vi "F510-X.vi"(8 "error in (no error)":errorcluster, 10 "Deadzone Scale Cluster":cluster{"Scale":dbl, "Deadzone":dbl}={"Scale"=1.0, "Deadzone"=0.1}, 11 "refnum name":string) -> (0 "error out":errorcluster, 1 "Right Stick":cluster{"X":dbl, "Y":dbl}, 2 "Left Stick":cluster{"X":dbl, "Y":dbl}, 3 "JoystickDevRef":T2, 4 "Buttons":T1, 5 "Triggers":cluster{"Left":dbl, "Right":dbl}, 6 "D-Pad Buttons":T4)   [LabVIEW 2016]
uses:
  <vilib>/Rock Robotics/WPI/Joystick/WPI_JoystickDevRef.ctl
  <vilib>/Rock Robotics/WPI/Joystick/WPI_JoystickDeviceEnum.ctl
  <vilib>/Rock Robotics/WPI/Utilities/WPI_GetSetVariantRefNum.vi
panel:
  in  "Smooth Control (T)":bool=TRUE
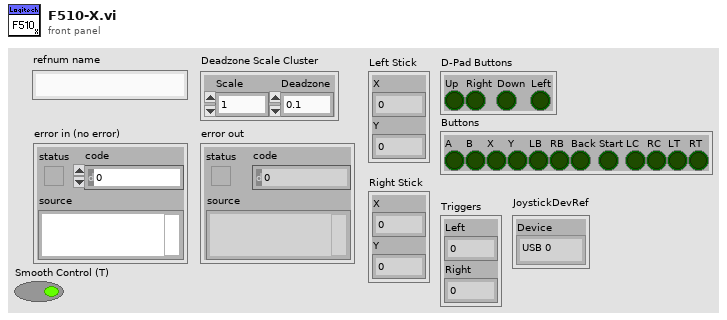
[diagram p1: front panel]
types:
  T1 = cluster{"A":bool, "B":bool, "X":bool, "Y":bool, "LB":bool, "RB":bool, "Back":bool, "Start":bool, "LC":bool, "RC":bool, "LT":bool, "RT":bool}
  T2 = typedef "WPI_JoystickDevRef.ctl" = cluster{"Device":T3}
  T3 = typedef "WPI_JoystickDeviceEnum.ctl" = enum16{"USB 0", "USB 1", "USB 2", "USB 3", "USB 4", "USB 5"}
  T4 = cluster{"Up":bool, "Right":bool, "Down":bool, "Left":bool}
  T5 = cluster{"[0]":dbl, "[1]":dbl, "[2]":dbl, "[3]":dbl, "[4]":dbl, "[5]":dbl}
  T6 = cluster{"Buttons[0]":bool, "Buttons[1]":bool, "Buttons[2]":bool, "Buttons[3]":bool, "Buttons[4]":bool, "Buttons[5]":bool, "Buttons[6]":bool, "Buttons[7]":bool, "Buttons[8]":bool, "Buttons[9]":bool}
  T7 = cluster{"Up":bool, "Down":bool, "Left":bool, "Right":bool}[]
  T8 = cluster{"Up":bool, "Down":bool, "Left":bool, "Right":bool}
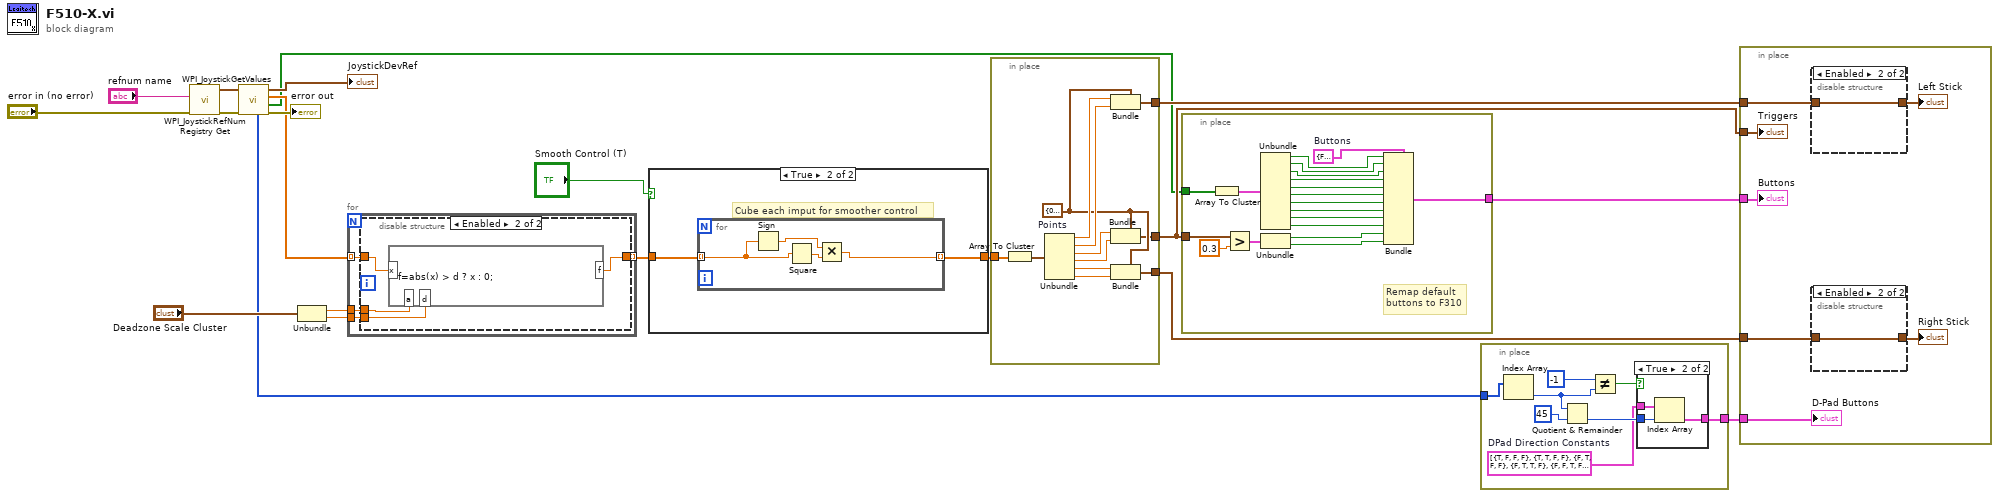
[diagram p0: block diagram]
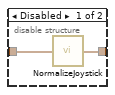
[diagram p3: hidden frame]
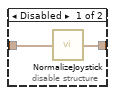
[diagram p4: hidden frame]
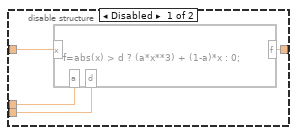
[diagram p6: hidden frame]
diagram:
  n1 = call <vilib>:"WPI_JoystickRefNum Registry Get.vi"("error in (no error)"="error in (no error)", "refnum name"="refnum name") -> ("error out"=w17:errorcluster, "JoystickDevRef"=w18:T2)  [unwired: 8 in]
  n2 = call <vilib>:"WPI_JoystickGetValues.vi"("error in (no error)"=w17, "JoystickDevRef"=w18) -> ("error out"=→"error out":errorcluster, "Buttons"=w5:bool[], "Axes"=w15:dbl[], "JoystickDevRef"=→"JoystickDevRef":T2, "POVs"=w9:i16[])  [unwired: 5 in]
  n3 = Unbundle("Deadzone Scale Cluster") -> ("Scale"=w13:dbl, "Deadzone"=w12:dbl)
  n4 = for {
    tunnel: w15 -> [w24] mode=indexing
    tunnel: w13 -> [w23]
    tunnel: w12 -> [w22]
    tunnel: [w21] -> w1 mode=indexing
    n5 = disable-structure shown="Enabled" {
      disable-tunnel: w24 -> [w28 w30]
      disable-tunnel: w23 -> [w27 w32]
      disable-tunnel: w22 -> [w26 w31]
      disable-tunnel: [w25 w29] -> w21
      frame Disabled {
        n6 = formula code="f=abs(x) > d ? (a*x**3) + (1-a)*x : 0;"("x"=w28, "d"=w26, "a"=w27) -> ("f"=w25:dbl)
      }
      frame Enabled {
        n7 = formula code="f=abs(x) > d ? x : 0;"("x"=w30, "d"=w31, "a"=w32) -> ("f"=w29:dbl)
      }
    }
  }
  n8 = case shown="True" "Smooth Control (T)" {
    tunnel: [w33 w34] -> w2
    tunnel: w1 -> [w33 w35]
    frame False {
    }
    frame True {
      # "Cube each imput for smoother control"
      n9 = for {
        tunnel: w35 -> [w37] mode=indexing
        tunnel: [w38] -> w34 mode=indexing
        n10 = Sign(1:w37) -> (0:w36:dbl)
        n11 = Square(x=w37) -> (x^2=w39:dbl)
        n12 = Multiply(x=w36, y=w39) -> (x*y=w38:dbl)
      }
    }
  }
  n13 = in-place {
    in-place-border: w2 -> [w48]
    in-place-border: [w44] -> w10
    in-place-border: [w47] -> w11
    in-place-border: [w42] -> w8
    w43 = cluster{"X":dbl, "Y":dbl} {"X"=0.0, "Y"=0.0}  # Points
    n14 = Array To Cluster(array=w48) -> (cluster=w51:T5)
    n15 = Unbundle(w51) -> ("[0]"=w49:dbl, "[1]"=w50:dbl, "[2]"=w41:dbl, "[3]"=w40:dbl, "[4]"=w46:dbl, "[5]"=w45:dbl)
    n16 = Bundle(cluster=w43, "X"=w49, "Y"=w50) -> (w47:cluster{"X":dbl, "Y":dbl})
    n17 = Bundle(cluster=w43, "X"=w41, "Y"=w40) -> (w42:cluster{"X":dbl, "Y":dbl})
    n18 = Bundle(cluster=w43, "X"=w46, "Y"=w45) -> (w44:cluster{"X":dbl, "Y":dbl})
  }
  n19 = in-place {
    in-place-border: w5 -> [w61]
    in-place-border: [w63] -> w4
    in-place-border: w8 -> [w56]
    w70 = T1 {"A"=FALSE, "B"=FALSE, "X"=FALSE, "Y"=FALSE, "LB"=FALSE, "RB"=FALSE, "Back"=FALSE, "Start"=FALSE, "LC"=FALSE, "RC"=FALSE, "LT"=FALSE, "RT"=FALSE}  # Buttons
    # "Remap default\nbuttons to F310"
    n20 = Array To Cluster(array=w61) -> (cluster=w62:T6)
    n21 = Greater?(x=w56, y=0.3) -> (0:w54:cluster{"X":bool, "Y":bool})
    n22 = Unbundle(w62) -> ("Buttons[0]"=w69:bool, "Buttons[1]"=w68:bool, "Buttons[2]"=w67:bool, "Buttons[3]"=w66:bool, "Buttons[4]"=w65:bool, "Buttons[5]"=w64:bool, "Buttons[6]"=w60:bool, "Buttons[7]"=w59:bool, "Buttons[8]"=w58:bool, "Buttons[9]"=w57:bool)
    n23 = Unbundle(w54) -> ("X"=w53:bool, "Y"=w52:bool)
    n24 = Bundle(cluster=w70, "A"=w69, "B"=w68, "X"=w67, "Y"=w66, "LB"=w65, "RB"=w64, "Back"=w60, "Start"=w59, "LC"=w58, "RC"=w57, "LT"=w53, "RT"=w52) -> (w63:T1)
  }
  n25 = in-place {
    in-place-border: w9 -> [w78]
    in-place-border: [w73] -> w7
    w74 = T7 [{"Up"=TRUE, "Down"=FALSE, "Left"=FALSE, "Right"=FALSE}, {"Up"=TRUE, "Down"=TRUE, "Left"=FALSE, "Right"=FALSE}, {"Up"=FALSE, "Down"=TRUE, "Left"=FALSE, "Right"=FALSE}, {"Up"=FALSE, "Down"=TRUE, "Left"=TRUE, "Right"=FALSE}, {"Up"=FALSE, "Down"=FALSE, "Left"=TRUE, "Right"=FALSE}, {"Up"=FALSE, "Down"=FALSE, "Left"=TRUE, "Right"=TRUE}, {"Up"=FALSE, "Down"=FALSE, "Left"=FALSE, "Right"=TRUE}, {"Up"=TRUE, "Down"=FALSE, "Left"=FALSE, "Right"=TRUE}]  # DPad Direction Constants
    n26 = Index Array(array=w78) -> (element=w72:i16)  [unwired: 1 in]
    n27 = Quotient & Remainder(x=w72, y=u16 45) -> (floor(x/y)=w76:u16)  [unwired: 1 out]
    n28 = Not Equal?(x=i16 -1, y=w72) -> (x != y?=w75:bool)
    n29 = case shown="True" w75 {
      tunnel: w76 -> [_ w81]
      tunnel: w74 -> [_ w80]
      tunnel: [_ w79] -> w73
      frame False {
      }
      frame True {
        n30 = Index Array(array=w80, index=w81) -> (element=w79:T8)
      }
    }
  }
  n31 = in-place {
    in-place-border: w11 -> [w85]
    in-place-border: w10 -> [w83]
    in-place-border: w8 -> [w88]
    in-place-border: w7 -> [w87]
    in-place-border: w4 -> [w86]
    n32 = disable-structure shown="Enabled" {
      disable-tunnel: w85 -> [w93 w94]
      disable-tunnel: [w92 w94] -> w84
      frame Disabled {
        n33 = call "NormalizeJoystick.vi"("joystick"=w93) -> ("normalized joystick"=w92:cluster{"x":dbl, "y":dbl})
      }
      frame Enabled {
      }
    }
    "Left Stick" <- w84
    n34 = disable-structure shown="Enabled" {
      disable-tunnel: w83 -> [w90 w91]
      disable-tunnel: [w89 w91] -> w82
      frame Disabled {
        n35 = call "NormalizeJoystick.vi"("joystick"=w90) -> ("normalized joystick"=w89:cluster{"x":dbl, "y":dbl})
      }
      frame Enabled {
      }
    }
    "Right Stick" <- w82
    "Triggers" <- w88
    "D-Pad Buttons" <- w87
    "Buttons" <- w86
  }
